vi "Evaluator_Init.vi"(0 "object in":refnum<class "Evaluator.lvclass">, 5 "error in (no error)":errorcluster) -> (14 "object out":refnum<class "Evaluator.lvclass">, 19 "error out":errorcluster)   [LabVIEW 2023, in "Evaluator.lvclass"]
uses:
  Evaluator.lvclass
  Evaluator.lvclass/Evaluator.ctl
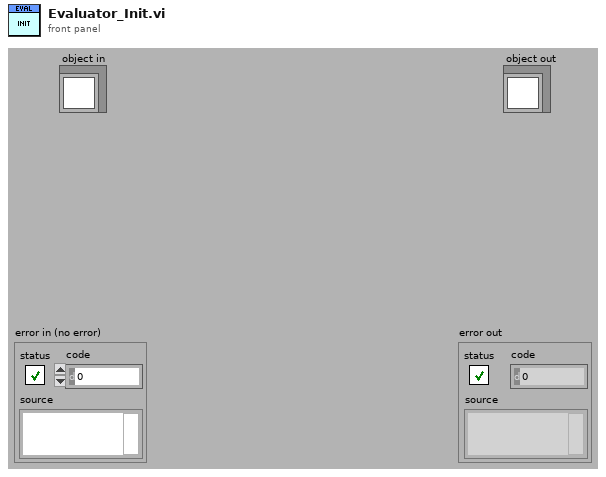
[diagram p1: front panel]
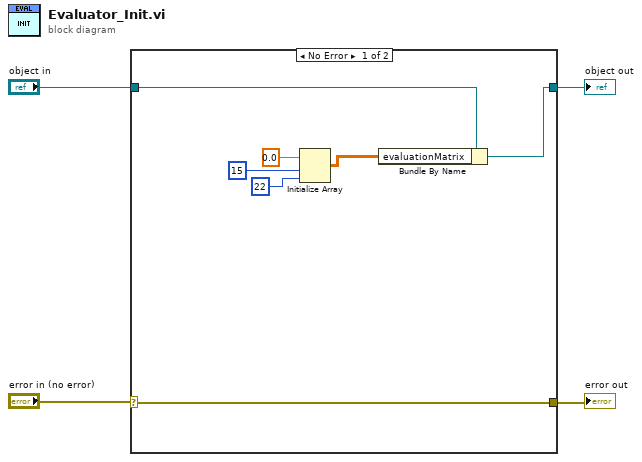
[diagram p0: block diagram]
diagram:
  n1 = case shown="No Error" "error in (no error)" {
    selector: "error in (no error)" -> [w11 w12]
    tunnel: "object in" -> [w10 w13]
    tunnel: [w5 w13] -> w3
    tunnel: [w11 w12] -> w1
    frame No Error {
      n2 = Initialize Array(0.0 ("element"), 15 ("dimension size"), 22 ("dimension size")) -> (w6:dbl[][])
      n3 = Bundle By Name(cluster=w10, "evaluationMatrix"=w6) -> (w5:refnum<class "Evaluator.lvclass">)
    }
    frame Error {
    }
  }
  "object out" <- w3
  "error out" <- w1
